vi "initialise.vi"(8 "error in (no error)":errorcluster, 11 "ScanModeMG090624Camera in":refnum<class "ImagingModeMG090624Camera.lvclass">) -> (0 "error out":errorcluster, 3 "ScanModeMG090624Camera out":refnum<class "ImagingModeMG090624Camera.lvclass">)   [LabVIEW 2010, in "ImagingModeMG090624Camera.lvclass"]
doc: "The dynamic dispatch-version of this VI initalises the plug-in object by allocating and initalising any dynamic resources need."
uses:
  ImagingModeMG090624Camera.lvclass
  ImagingModeDL091001Scaffold/ImagingModeDL091001Scaffold/ImagingModeDL091001Scaffold.lvclass
  Instrument/GenericInstrument/GenericInstrument/GenericInstrument.lvclass
  ScanHead/GenericScanHead/GenericScanHead/GenericScanHead.lvclass
  Display/GenericDisplay/GenericDisplay/GenericDisplay.lvclass
  Stimulator/GenericStimulator/GenericStimulator/GenericStimulator.lvclass
  Analyser/GenericAnalyser/GenericAnalyser/GenericAnalyser.lvclass
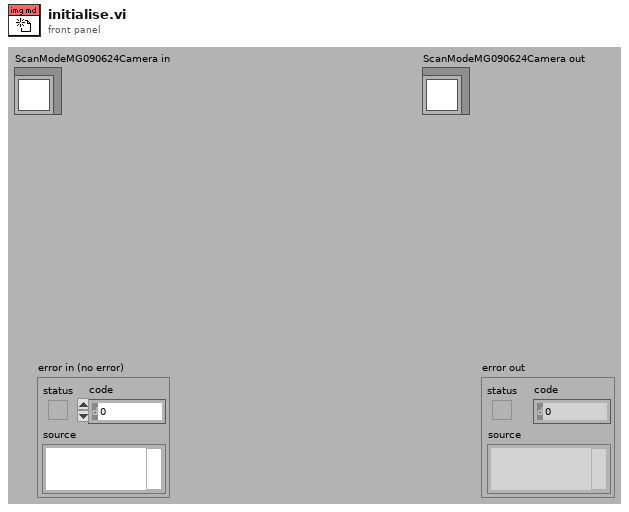
[diagram p1: front panel]
types:
  T1 = typedef "controls_refs.ctl" = cluster{"scan start button":refnum<vi>, "tabs":cluster{"main":refnum<vi>, "settings":refnum<vi>}, "subpanels":cluster{"imagingMode":refnum<vi>, "scanHead":refnum<vi>, "display":refnum<vi>, "experimentController":refnum<vi>, "instrument":refnum<vi>, "stage":refnum<vi>, "stimulator":refnum<vi>, "dataCollection":refnum<vi>, "analyser":refnum<vi>, "daq":refnum<vi>, "imageAssembler":refnum<vi>}, "drop-downs":cluster{"run mode":refnum<vi>, "imagingMode":refnum<vi>, "experimentalController":refnum<vi>, "objective":refnum<vi>}, "status lights":cluster{"experimentController":refnum<vi>, "imagingMode":refnum<vi>, "scanHead":refnum<vi>, "daq":refnum<vi>, "imageAssembler":refnum<vi>, "dataCollection":refnum<vi>, "display":refnum<vi>, "analyser":refnum<vi>, "stage":refnum<vi>, "stimulator":refnum<vi>, "instrument":refnum<vi>}, "message":refnum<vi>, "stimulator enabled?":refnum<vi>, "saving":cluster{"data folder path":refnum<vi>, "file base name":refnum<vi>, "notebook":refnum<vi>}, "progress bar":refnum<vi>, "update icon":refnum<vi>, "title":refnum<vi>, "main vi":refnum<vi>, "user":refnum<vi>, "exit_button":refnum<vi>, "CPU usage %":refnum<vi>}
  T2 = typedef "GenericToplevelComponent.lvclass/common_trigger_enum.ctl" = enum16{"NULL", "initialise", "terminate", "fetch command", "fetch data", "attach observer", "register as observer", "detach observer", "acknowledge", "start", "stop", "sweep started", "sweep finished", "experiment started", "experiment stopped"}
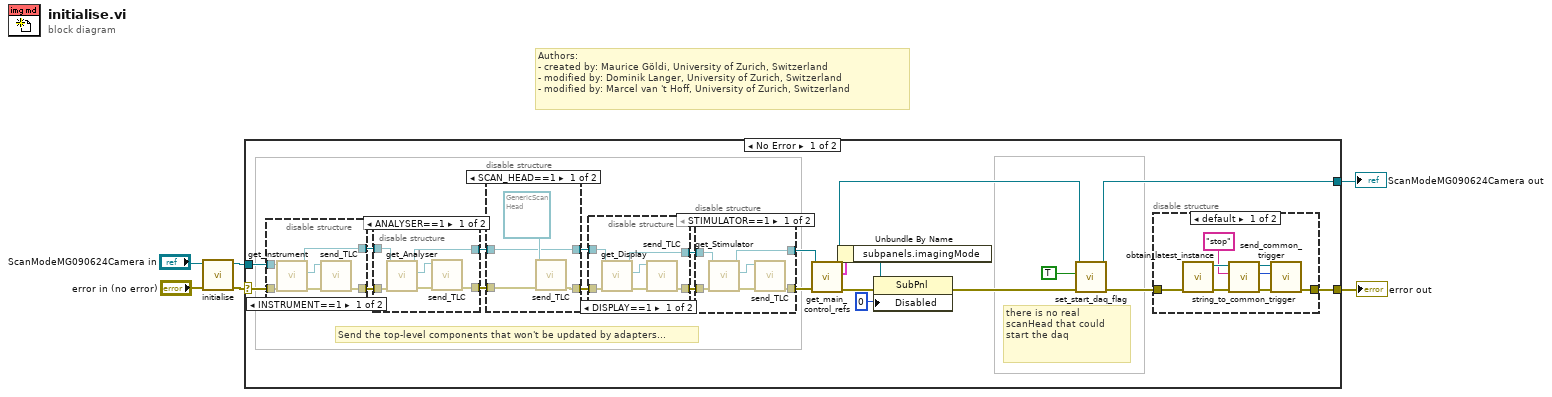
[diagram p0: block diagram]
diagram:
  # "Authors: \n- created by: Maurice Göldi, University of Zurich, Switzerland\n- modified by: Dominik Langer, University of Zurich, Switzerland\n- modified by: Marcel van 't Hoff, University of Zurich, Switzerland"
  n1 = call-parent "initialise.vi"("error in (no error)"="error in (no error)", "GenericPlugin in"="ScanModeMG090624Camera in") -> ("error out"=w3:errorcluster, "GenericPlugin out"=w4:refnum<class "ImagingModeMG090624Camera.lvclass">)  [unwired: 8 out]
  n2 = case shown="No Error" w3 {
    selector: w3 -> [w19 w77]
    tunnel: [w8 w77] -> w5
    tunnel: [w7 w76] -> w2
    tunnel: w4 -> [w16 w76]
    frame No Error {
      # "there is no real scanHead that could start the daq"
      # "Send the top-level components that won't be updated by adapters..."
      n3 = disable-structure shown="INSTRUMENT==1" {
        disable-tunnel: w19 -> [w63 w66]
        disable-tunnel: w16 -> [w62 w65]
        disable-tunnel: [w60 w66] -> w14
        disable-tunnel: [w59 w65] -> w13
        frame condition #0 {
          n4 = call-dynamic "get_Instrument.vi"("error in (no error)"=w63, "ScanModeDL090923Scaffold in"=w62) -> ("error out"=w64:errorcluster, "Instrument"=w61:refnum<class "GenericInstrument.lvclass">, "ScanModeDL090923Scaffold out"=w59:refnum<class "ImagingModeMG090624Camera.lvclass">)  [unwired: 4 in, 3 out]
          n5 = call-dynamic "send_TLC.vi"("error in (no error)"=w64, "GenericToplevelComponent in"=w61) -> ("error out"=w60:errorcluster)  [unwired: 8 in, 1 out]
        }
        frame condition #1 (active) {
        }
      }
      n6 = disable-structure shown="ANALYSER==1" {
        disable-tunnel: [w56 w58] -> w20
        disable-tunnel: [w54 w57] -> w17
        disable-tunnel: w14 -> [w52 w58]
        disable-tunnel: w13 -> [w51 w57]
        frame condition #0 {
          n7 = call-dynamic "get_Analyser.vi"("error in (no error)"=w52, "ScanModeDL090923Scaffold in"=w51) -> ("error out"=w55:errorcluster, "Analyser"=w53:refnum<class "GenericAnalyser.lvclass">, "ScanModeDL090923Scaffold out"=w54:refnum<class "ImagingModeMG090624Camera.lvclass">)  [unwired: 4 in, 3 out]
          n8 = call-dynamic "send_TLC.vi"("error in (no error)"=w55, "GenericToplevelComponent in"=w53) -> ("error out"=w56:errorcluster)  [unwired: 8 in, 1 out]
        }
        frame condition #1 (active) {
        }
      }
      n9 = disable-structure shown="SCAN_HEAD==1" {
        disable-tunnel: w20 -> [w47 w49]
        disable-tunnel: [w48 w49] -> w18
        disable-tunnel: w17 -> [w45 w50]
        disable-tunnel: [w45 w50] -> w15
        frame condition #0 {
          n10 = call-dynamic "send_TLC.vi"("error in (no error)"=w47, "GenericToplevelComponent in"=refnum<class "GenericScanHead.lvclass"> refnum ("GenericScanHead.lvclass")) -> ("error out"=w48:errorcluster)  [unwired: 8 in, 1 out]
        }
        frame condition #1 (active) {
        }
      }
      n11 = disable-structure shown="DISPLAY==1" {
        disable-tunnel: [w40 w43] -> w24
        disable-tunnel: [w39 w44] -> w22
        disable-tunnel: w18 -> [w38 w44]
        disable-tunnel: w15 -> [w37 w43]
        frame condition #0 {
          n12 = call-dynamic "get_Display.vi"("error in (no error)"=w38, "ScanModeDL090923Scaffold in"=w37) -> ("error out"=w41:errorcluster, "Display"=w42:refnum<class "GenericDisplay.lvclass">, "ScanModeDL090923Scaffold out"=w40:refnum<class "ImagingModeMG090624Camera.lvclass">)  [unwired: 7 out]
          n13 = call-dynamic "send_TLC.vi"("error in (no error)"=w41, "GenericToplevelComponent in"=w42) -> ("error out"=w39:errorcluster)  [unwired: 8 in, 1 out]
        }
        frame condition #1 (active) {
        }
      }
      n14 = disable-structure shown="STIMULATOR==1" {
        disable-tunnel: w24 -> [w34 w36]
        disable-tunnel: [w33 w36] -> w23
        disable-tunnel: w22 -> [w32 w35]
        disable-tunnel: [w30 w35] -> w21
        frame condition #0 {
          n15 = call-dynamic "get_Stimulator.vi"("error in (no error)"=w32, "ScanModeDL090923Scaffold in"=w34) -> ("error out"=w31:errorcluster, "Stimulator"=w29:refnum<class "GenericStimulator.lvclass">, "ScanModeDL090923Scaffold out"=w33:refnum<class "ImagingModeMG090624Camera.lvclass">)  [unwired: 4 in, 3 out]
          n16 = call-dynamic "send_TLC.vi"("error in (no error)"=w31, "GenericToplevelComponent in"=w29) -> ("error out"=w30:errorcluster)  [unwired: 8 in, 1 out]
        }
        frame condition #1 (active) {
        }
      }
      n17 = call-dynamic "get_main_control_refs.vi"("error in (no error)"=w21, "GenericPlugin.lvclass in"=w23) -> ("error out"=w26:errorcluster, "control references"=w28:T1, "GenericPlugin.lvclass out"=w10:refnum<class "ImagingModeMG090624Camera.lvclass">)  [unwired: 7 out]
      n18 = Unbundle By Name(w28) -> ("subpanels.imagingMode"=w27:refnum<vi>)
      n19 = property class="SubPnl"(reference=w27, error in=w26, "Disabled"=u8 0) -> (error out=w12:errorcluster)  [unwired: 1 out]
      n20 = call-dynamic "set_start_daq_flag.vi"("error in (no error)"=w12, "start daq from within imagingMode?"=TRUE, "ImagingModeDL090923Scaffold in"=w10) -> ("error out"=w9:errorcluster, "ImagingModeDL090923Scaffold out"=w7:refnum<class "ImagingModeMG090624Camera.lvclass">)  [unwired: 7 in]
      n21 = disable-structure shown="default" {
        disable-tunnel: w9 -> [w74 w75]
        disable-tunnel: [w73 w75] -> w8
        frame condition #0 (active) {
          n22 = call "obtain_latest_instance.vi"("error in (no error)"=w74) -> ("error out"=w70:errorcluster, "microscope"=w72:refnum<class "GenericInstrument.lvclass">)  [unwired: 9 in]
          n23 = call-dynamic "string_to_common_trigger.vi"("error in (no error)"=w70, "trigger string"="stop", "GenericToplevelComponent in"=w72) -> ("error out"=w69:errorcluster, "trigger"=w67:T2, "GenericToplevelComponent out"=w71:refnum<class "GenericInstrument.lvclass">)  [unwired: 6 in]
          n24 = call-dynamic "send_common_trigger.vi"("error in (no error)"=w69, "trigger"=w67, "GenericToplevelComponent in"=w71) -> ("error out"=w73:errorcluster)  [unwired: 6 in, 2 out]
        }
        frame condition #1 {
        }
      }
    }
    frame Error {
    }
  }
  "error out" <- w5
  "ScanModeMG090624Camera out" <- w2
